vi "C to K.vi"(11 "Temperature (C)":dbl) -> (3 "Temperature (K)":dbl)   [LabVIEW 2019]
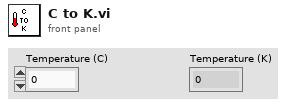
[diagram p1: front panel]
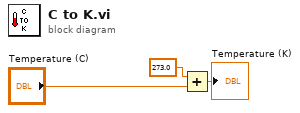
[diagram p0: block diagram]
diagram:
  n1 = Add(x=273.0, y="Temperature (C)") -> (x+y=→"Temperature (K)":dbl)
